vi "Set Vecto.vi"(10 "Vecto":refnum<class "Vecto.lvclass">, 11 "VolatusAPI in":refnum<class "VolatusAPI.lvclass">) -> (3 "VolatusAPI out":refnum<class "VolatusAPI.lvclass">)   [LabVIEW 2020, in "Volatus.lvlib" / "VolatusAPI.lvclass"]
uses:
  VolatusAPI.lvclass
  lv-vecto/Vecto/Vecto/Vecto.lvclass
  VolatusAPI.lvclass/VolatusAPI.ctl
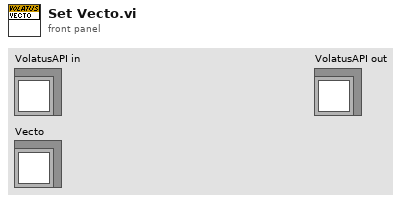
[diagram p1: front panel]
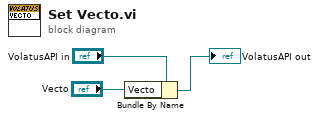
[diagram p0: block diagram]
diagram:
  n1 = Bundle By Name(cluster="VolatusAPI in", "Vecto"="Vecto") -> (→"VolatusAPI out":refnum<class "VolatusAPI.lvclass">)
